vi "test-ltv-differential-drive-controller-Test1.vi"() -> (3 "All tests passed":bool)   [LabVIEW 2019]
uses:
  <vilib>/Rock Robotics/WPI/ThirdParty/JAS_Junk/TrajLib/TRAJ_STATE.ctl
  <vilib>/Rock Robotics/WPI/ThirdParty/JAS_Junk/TrajLib/POSE2D.ctl
  <vilib>/Rock Robotics/WPI/ThirdParty/JAS_Junk/TrajLib/TRANSLATION2D.ctl
  <vilib>/Rock Robotics/WPI/ThirdParty/JAS_Junk/TrajLib/ROTATION2D.ctl
  <vilib>/Rock Robotics/WPI/ThirdParty/JAS_Junk/TrajLib/LINEAR_SYSTEM.ctl
  <vilib>/Analysis/Matrix/Datatypes/RealMatrix.ctl
  <vilib>/Rock Robotics/WPI/ThirdParty/JAS_Junk/TrajLib/LTV_DIFF_DRIVE_CTRL.ctl
  <vilib>/Rock Robotics/WPI/ThirdParty/JAS_Junk/TrajLib/FUNCTION_GENERATOR_MATRIX.ctl
  <vilib>/Rock Robotics/WPI/ThirdParty/JAS_Junk/TrajLib/TRAJECTORY_SPLINE_TYPE_ENUM.ctl
  <vilib>/numeric/Random Number (Range) DBL.vi
  <vilib>/Rock Robotics/WPI/ThirdParty/JAS_Junk/TrajLib/Conv_Inches_Meters.vi
  <vilib>/Rock Robotics/WPI/ThirdParty/JAS_Junk/TrajLib/Rotation2d_CreateAngle.vi
  <vilib>/Rock Robotics/WPI/ThirdParty/JAS_Junk/TrajLib/Translation2d_Create.vi
  <vilib>/Rock Robotics/WPI/ThirdParty/JAS_Junk/TrajLib/MatBuilder_Create.vi
  <vilib>/Rock Robotics/WPI/ThirdParty/JAS_Junk/TrajLib/LinearSystem_New.vi
  <vilib>/Rock Robotics/WPI/ThirdParty/JAS_Junk/TrajLib/MatrixHelper_Zero.vi
  <vilib>/Rock Robotics/WPI/ThirdParty/JAS_Junk/TrajLib/MatBuilder_Fill.vi
  <vilib>/Rock Robotics/WPI/ThirdParty/JAS_Junk/TrajLib/SlewRateLimiter_New.vi
  <vilib>/Rock Robotics/WPI/ThirdParty/JAS_Junk/TrajLib/SlewRateLimiter_Reset.vi
  <vilib>/Rock Robotics/WPI/ThirdParty/JAS_Junk/TrajLib/SlewRateLimiter_Calculate.vi
  <vilib>/Rock Robotics/WPI/ThirdParty/JAS_Junk/TrajLib/SlewRateLimiter_SetRate.vi
  <vilib>/Rock Robotics/WPI/ThirdParty/JAS_Junk/TrajLib/MatrixHelper_CoerceSize.vi
  <vilib>/Rock Robotics/WPI/ThirdParty/JAS_Junk/TrajLib/Util_GetTime.vi
  <vilib>/Rock Robotics/WPI/ThirdParty/JAS_Junk/TrajLib/Trajectory_Library.lvlib
  <vilib>/Analysis/Matrix/NI_Matrix.lvlib
panel:
  out "DiffDriveCtrl":T1
  out "Output":T3
  out "Return X":T3
  out "Time":dbl=-1.0
  out "Create Error":bool
  out "Linearsystem":T4
  out "Error":bool
  out "IterationCount":i32
  out "Any Calc Error":bool
  out "Waveform Graph":dbl[][](graph)
  out "XY Graph":cluster{dbl[], dbl[]}[](graph)
  out "X":bool
  out "Y":bool
  out "Rot":bool
  out "TotalTime_Sec":dbl
  out "Calc Error":bool
  out "TrajStatePose":T5={"TRANSLATION"={"X"=0.0, "Y"=0.0}, "ROTATION"={"VALUE"=0.0, "COS"=1.0, "SIN"=0.0}} {"ROTATION"."SIN" format="%13.4f"; "ROTATION"."COS" format="%13.4f"; "ROTATION"."VALUE" format="%13.4f"; "TRANSLATION"."Y" format="%14.3f"; "TRANSLATION"."X" format="%14.3f"}
  out "UpdatedPose":T5 {"ROTATION"."SIN" format="%13.4f"; "ROTATION"."COS" format="%13.4f"; "ROTATION"."VALUE" format="%13.4f"; "TRANSLATION"."Y" format="%14.3f"; "TRANSLATION"."X" format="%14.3f"}
  out "OutputTRAJ_STATE":T8={"TimeSeconds"=0.0, "Velocity"=0.0, "Acceleration"=0.0, "POSE"={"TRANSLATION"={"X"=0.0, "Y"=0.0}, "ROTATION"={"VALUE"=0.0, "COS"=1.0, "SIN"=0.0}}, "Curvature"=0.0} {"POSE"."ROTATION"."SIN" format="%13.4f"; "POSE"."ROTATION"."COS" format="%13.4f"; "POSE"."ROTATION"."VALUE" format="%13.4f"; "POSE"."TRANSLATION"."Y" format="%14.3f"; "POSE"."TRANSLATION"."X" format="%14.3f"}
  out "At Reference":bool
  in  "Use Noise":bool
  in  "Use Rate Limit":bool
  # "< 5, 1 >"
  # "< 2 1 >"
  # "<States,States>"
  # "<States,Inputs>"
  # "<Outputs,States>"
  # "<Outputs,Inputs>"
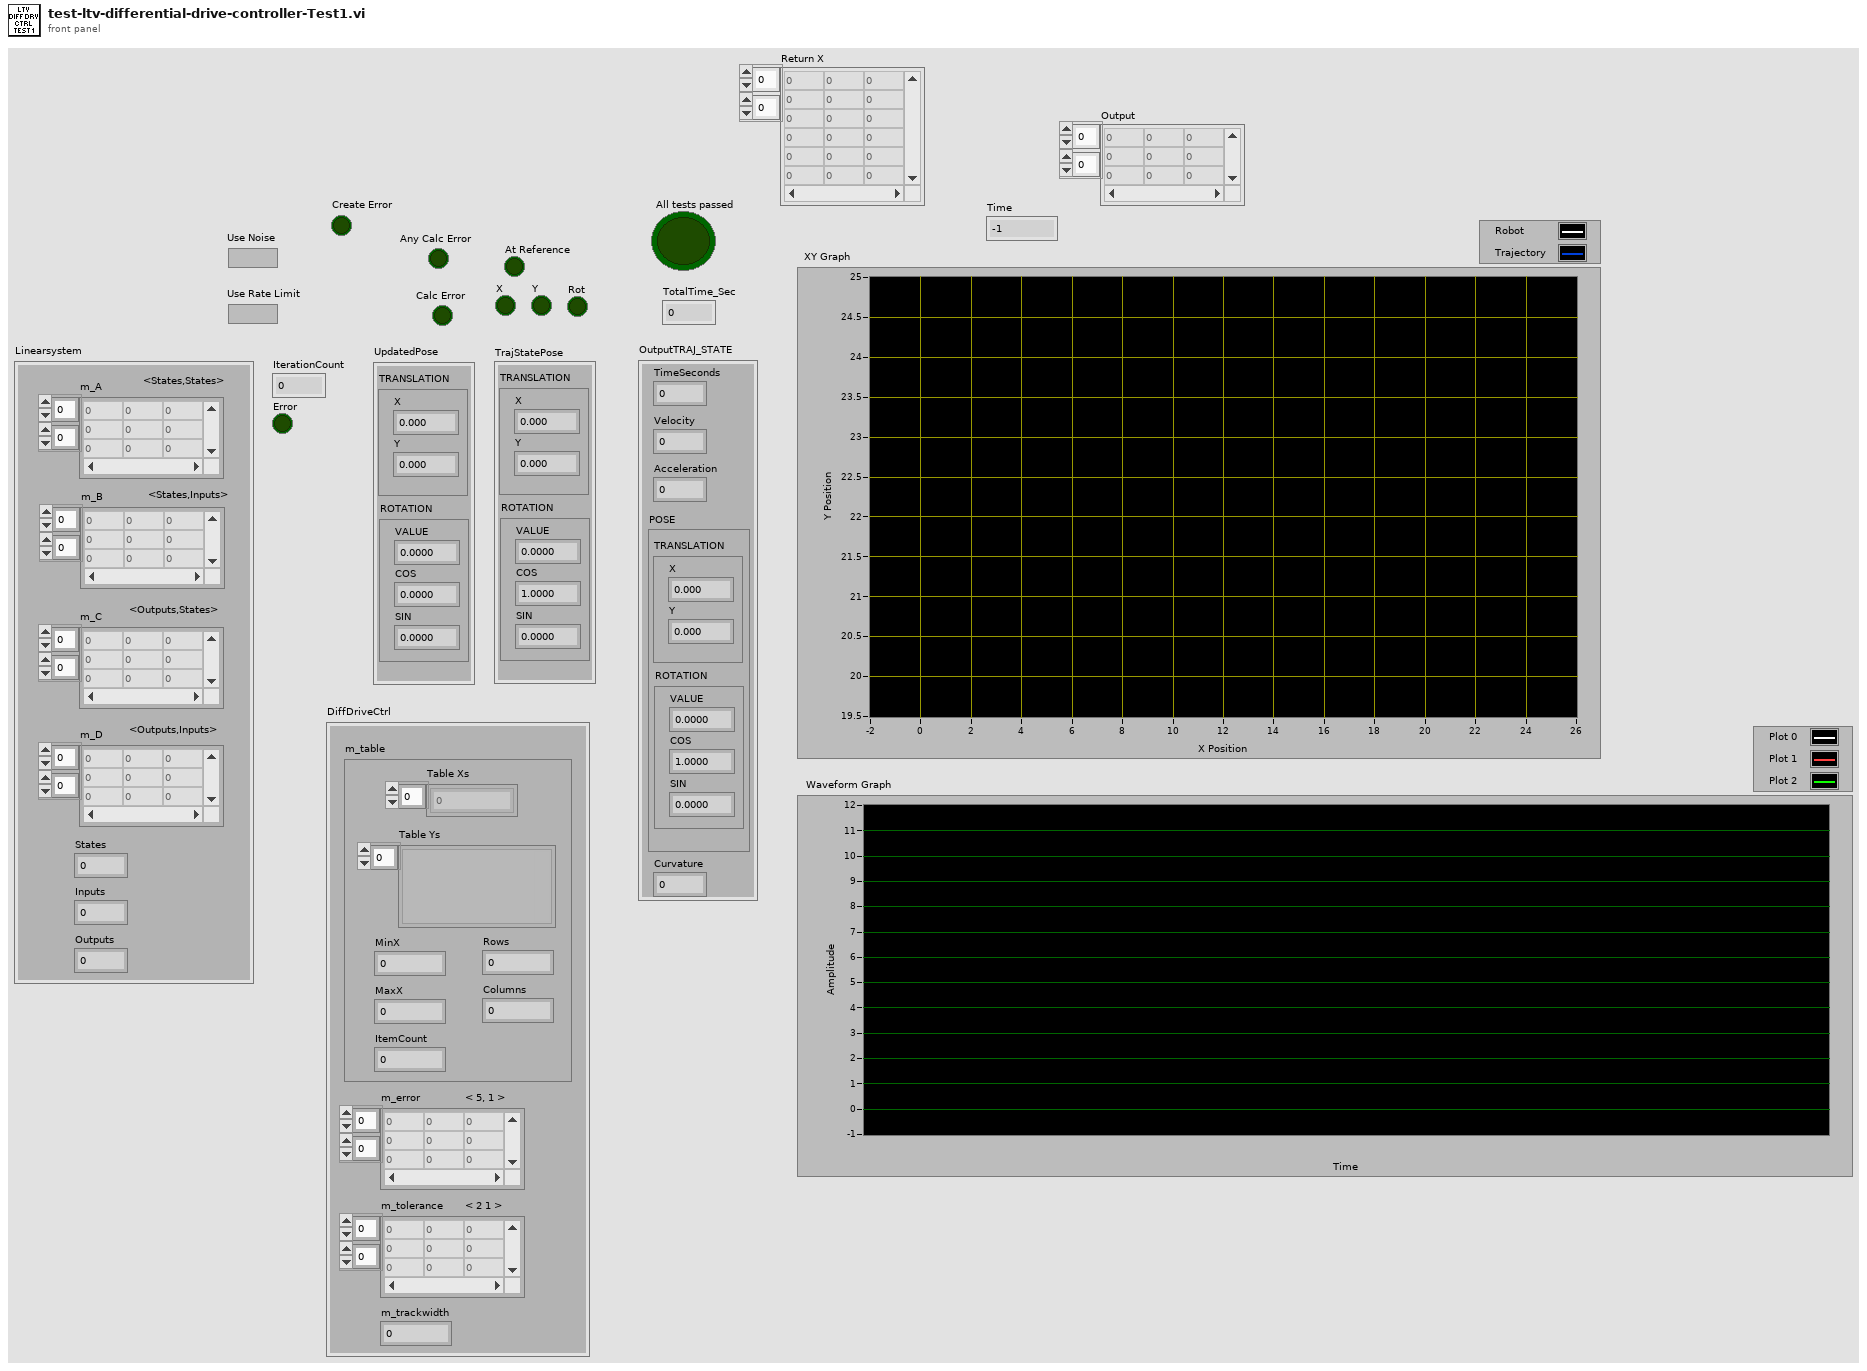
[diagram p1: front panel]
types:
  T1 = typedef "Trajectory_Library.lvlib/LTV_DIFF_DRIVE_CTRL.ctl" = cluster{"m_table":T2, "m_error":T3, "m_tolerance":T3, "m_trackwidth":dbl}
  T2 = typedef "Trajectory_Library.lvlib/FUNCTION_GENERATOR_MATRIX.ctl" = cluster{"Table Xs":dbl[], "Table Ys":variant[], "MinX":dbl, "MaxX":dbl, "ItemCount":i32, "Rows":i32, "Columns":i32}
  T3 = typedef "NI_Matrix.lvlib/RealMatrix.ctl" = dbl[][]
  T4 = typedef "Trajectory_Library.lvlib/LINEAR_SYSTEM.ctl" = cluster{"m_A":T3, "m_B":T3, "m_C":T3, "m_D":T3, "States":i32, "Inputs":i32, "Outputs":i32}
  T5 = typedef "Trajectory_Library.lvlib/POSE2D.ctl" = cluster{"TRANSLATION":T6, "ROTATION":T7}
  T6 = typedef "Trajectory_Library.lvlib/TRANSLATION2D.ctl" = cluster{"X":dbl, "Y":dbl}
  T7 = typedef "Trajectory_Library.lvlib/ROTATION2D.ctl" = cluster{"VALUE":dbl, "COS":dbl, "SIN":dbl}
  T8 = typedef "Trajectory_Library.lvlib/TRAJ_STATE.ctl" = cluster{"TimeSeconds":dbl, "Velocity":dbl, "Acceleration":dbl, "POSE":T5, "Curvature":dbl}
  T9 = typedef "Trajectory_Library.lvlib/TRAJECTORY_SPLINE_TYPE_ENUM.ctl" = enum16{"Cubic", "Cubic With Weights", "Quintic", "Quintic With Weights"}
  T10 = typedef "Trajectory_Library.lvlib/WEIGHTED_WAYPOINT.ctl" = cluster{"TRANSLATION":T6, "ROTATION":T7, "SCALAR":dbl}
  T11 = typedef "Trajectory_Library.lvlib/TRAJ_CONFIG.ctl" = cluster{"MaxVelocity":dbl, "Max Acceleration":dbl, "StartVelocity":dbl, "End Velocity":dbl, "Reversed":bool, "DiffDrKineConstntDefined":bool, "CentAcellConstntDefined":bool, "DiffDrVoltConstntDefined":bool, "DIFF_DRIVE_KINE_CONSTRAINT":T12, "CENTRIPETAL_ACCEL_CONSTRAINT":T14, "SwerveDrKineConstntDefined":bool, "SWERVE_DRIVE_KINE_CONSTRAINT":T15, "DIFF_DRIVE_VOLTAGE_CONSTRAINT":T17, "MECANUM_DRIVE_KINE_CONSTRAINT":T19, "MecanumDrKineConstntDefined":bool}
  T12 = typedef "Trajectory_Library.lvlib/TRAJ_CONSTRAINT_DIIF_DRIVE_KINEMATICS.ctl" = cluster{"Max Speed (M/S)":dbl, "DIFF_DRIVE_KINEMATICS":T13, "Max Accel (M/S2)":dbl}
  T13 = typedef "Trajectory_Library.lvlib/DIFF_DRIVE_KINEMATICS.ctl" = cluster{"TrackWidth_Meters":dbl}
  T14 = typedef "Trajectory_Library.lvlib/TRAJ_CONSTRAINT_CENTRIPETAL_ACCEL.ctl" = cluster{"Max Cent Accel":dbl}
  T15 = typedef "Trajectory_Library.lvlib/TRAJ_CONSTRAINT_SWERVE_DRIVE_KINEMATICS.ctl" = cluster{"Max Speed (M/S)":dbl, "SwerveKinematics":T16}
  T16 = typedef "Trajectory_Library.lvlib/SWERVE_DRIVE_KINEMATICS.ctl" = cluster{"NumModules":i32, "InverseKinematics":T3, "ForwardKinematics":T3, "Modules":T6[], "PrevCoR":T6}
  T17 = typedef "Trajectory_Library.lvlib/TRAJ_CONSTRAINT_DIIF_DRIVE_VOLTAGE.ctl" = cluster{"Max Voltage":dbl, "DIFF_DRIVE_KINEMATICS":T13, "SIMPLE_MOTOR_FF":T18}
  T18 = typedef "Trajectory_Library.lvlib/SIMPLE_MOTOR_FF.ctl" = cluster{"Ks":dbl, "Kv":dbl, "Ka":dbl}
  T19 = typedef "Trajectory_Library.lvlib/TRAJ_CONSTRAINT_MECA_DRIVE_KINEMATICS.ctl" = cluster{"Max Speed (M/S)":dbl, "MECA_DRIVE_KINEMATICS":T20}
  T20 = typedef "Trajectory_Library.lvlib/MECA_DRIVE_KINEMATICS.ctl" = cluster{"FrontLeft":T6, "FrontRight":T6, "RearLeft":T6, "RearRight":T6, "InverseKinematics":T3, "ForwardKinematics":T3, "PrevCoR":T6}
  T21 = typedef "Trajectory_Library.lvlib/TRAJECTORY.ctl" = cluster{"TotalTImeSecs":dbl, "States":T8[]}
  T22 = typedef "Trajectory_Library.lvlib/TWIST2D.ctl" = cluster{"dX":dbl, "dY":dbl, "dTHETA":dbl}
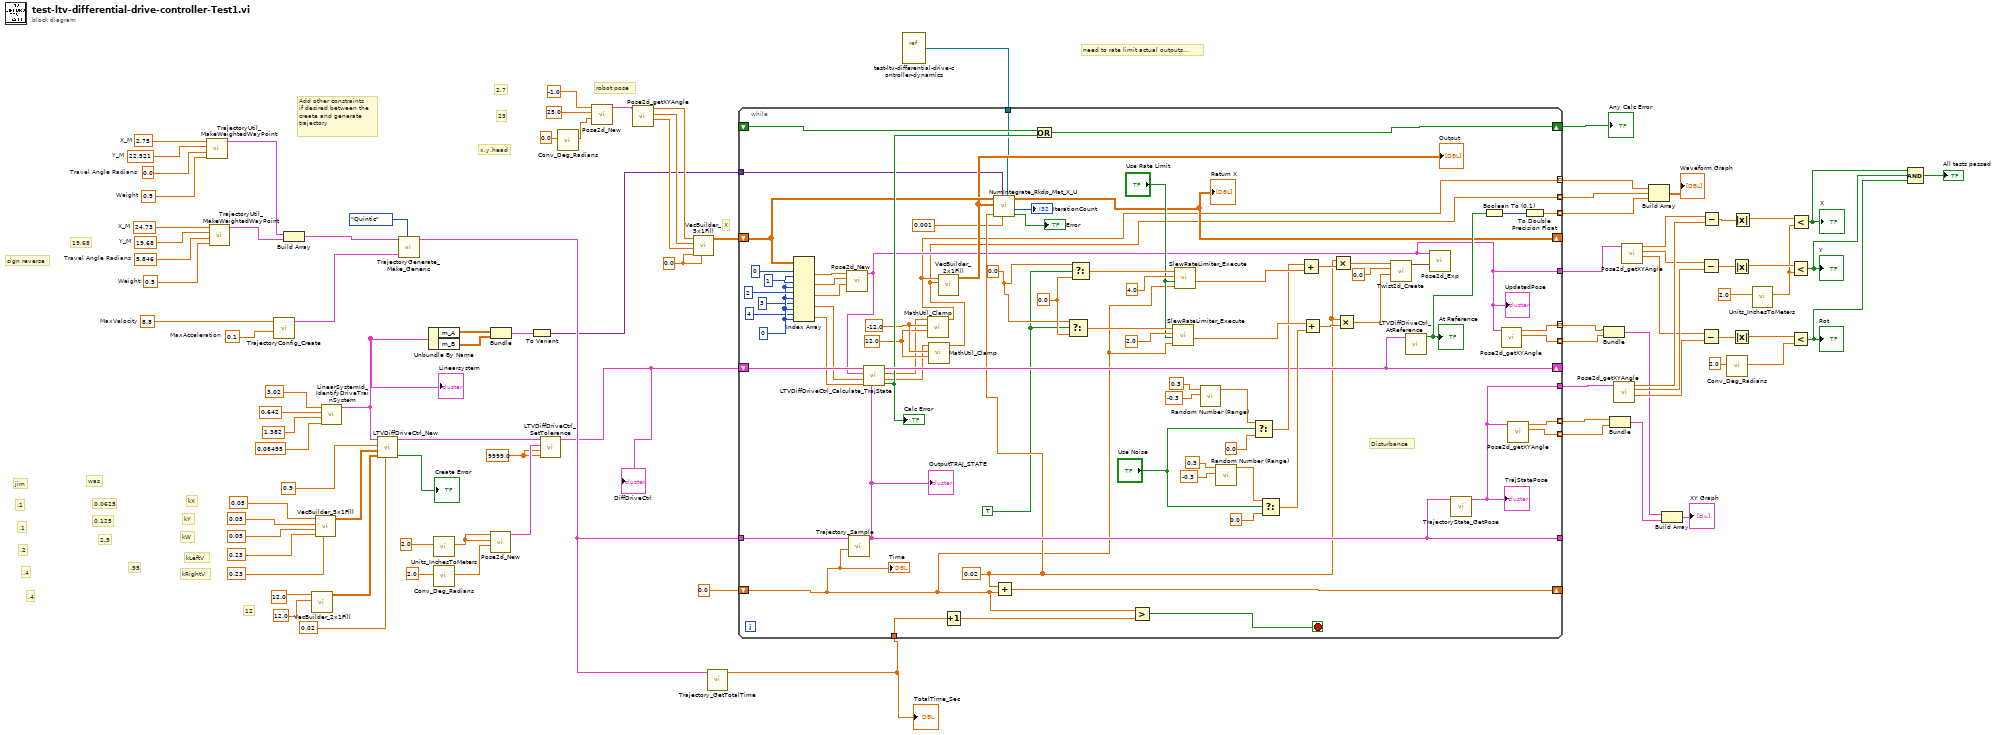
[diagram p0: block diagram]
diagram:
  w3 = 9999.0 ("LeftVelTolerance")
  w18 = 0.0 ("R3")
  w79 = 24.73  # X_M
  w78 = 19.68  # Y_M
  w66 = 5.846  # Travel Angle Radians
  w77 = 0.5  # Weight
  w76 = 2.75  # X_M
  w75 = 22.521  # Y_M
  w67 = 0.0  # Travel Angle Radians
  w74 = 0.5  # Weight
  w73 = 8.8  # MaxVelocity
  w72 = 0.1  # MaxAcceleration
  # ".4"
  # ".4"
  # ".2"
  # ".1"
  # ".1"
  # "jim"
  # "sign reverse"
  # "19.68"
  # ".95"
  # "12"
  # "need to rate limit actual outputs..."
  # "2.5"
  # "0.125"
  # "0.0625"
  # "was"
  # "X"
  # "23"
  # "2.7"
  # "x,y,head"
  # "robot pose"
  # "Add other constraints\nif desired between the\ncreate and generate\ntrajectory"
  # "kRightV"
  # "kLeftV"
  # "kW"
  # "kY"
  # "kX"
  n1 = call <vilib>:"TrajectoryUtil_MakeWeightedWayPoint.vi"("Weight"=w74, "Travel Angle Radians"=w67, "Y_M"=w75, "X_M"=w76) -> ("WEIGHTED_WAYPOINT"=w68:T10)  [unwired: 7 in]
  n2 = call <vilib>:"TrajectoryUtil_MakeWeightedWayPoint.vi"("Weight"=w77, "Travel Angle Radians"=w66, "Y_M"=w78, "X_M"=w79) -> ("WEIGHTED_WAYPOINT"=w80:T10)  [unwired: 7 in]
  n3 = call <vilib>:"TrajectoryConfig_Create.vi"("MaxAcceleration"=w72, "MaxVelocity"=w73) -> ("TRAJECTORY_CONFIG"=w71:T11)  [unwired: 9 in]
  n4 = Build Array(w68, w80) -> (w69:T10[])
  n5 = call <vilib>:"VecBuilder_2x1Fill.vi"("R1"=12.0, "R0"=12.0) -> ("output matrix"=w59:T3)  [unwired: 9 in]
  n6 = call <vilib>:"VecBuilder_5x1Fill.vi"("R4"=0.23, "R3"=0.23, "R2"=0.05, "R1"=0.05, "R0"=0.05) -> ("output matrix"=w60:T3)  [unwired: 6 in]
  n7 = call <vilib>:"LinearSystemId_IdentifyDriveTrainSystem.vi"("kAAngular"=0.08495, "kVAngular"=1.382, "kALinear"=0.642, "kVLinear"=3.02) -> ("Linearsystem"=w12:T4)  [unwired: 6 in, 1 out]
  "Linearsystem" <- w12
  n8 = call <vilib>:"LTVDiffDriveCtrl_New.vi"("dT"=0.02, "Relms"=w59, "Qelms"=w60, "TrackWidth"=0.9, "Plant"=w12) -> ("Error"=→"Create Error":bool, "DiffDriveCtrl"=w6:T1)  [unwired: 5 in]
  n9 = call <vilib>:"TrajectoryGenerate_Make_Generic.vi"("Spline Type"=TRAJECTORY_SPLINE_TYPE_ENUM."Quintic", "traj_config"=w71, "WeightedWayPoints"=w69) -> ("TRAJECTORY"=w56:T21)  [unwired: 7 in, 1 out]
  n10 = Unbundle By Name(w12) -> ("m_A"=w16:T3, "m_B"=w15:T3)
  n11 = call <vilib>:"Units_InchesToMeters.vi"("Inches"=2.0 ("x")) -> ("Meters"=w8:dbl)  [unwired: 10 in]
  n12 = call <vilib>:"Conv_Deg_Radians.vi"("Degress"=2.0) -> ("Radians"=w7:dbl)  [unwired: 10 in]
  n13 = call <vilib>:"Pose2d_New.vi"("Heading"=w7, "Y"=w8, "X"=w8) -> ("out POSe"=w4:T5)  [unwired: 8 in]
  n14 = Bundle("m_A"=w16, "m_B"=w15) -> (w14:cluster{"m_A":T3, "m_B":T3})  [unwired: 1 in]
  n15 = To Variant(anything=w14) -> (Variant=w13:variant)
  n16 = call <vilib>:"LTVDiffDriveCtrl_SetTolerance.vi"("RightVelTolerance"=w3, "LeftVelTolerance"=w3, "PoseTolerance"=w4, "in LTV_DIFF_DRIVE_CONTROLLER"=w6) -> ("out LTV_DIFF_DRIVE_CONTROLLER"=w5:T1)  [unwired: 7 in]
  "DiffDriveCtrl" <- w5
  n17 = call <vilib>:"Conv_Deg_Radians.vi"("Degress"=0.0) -> ("Radians"=w65:dbl)  [unwired: 10 in]
  n18 = call <vilib>:"Pose2d_New.vi"("Heading"=w65, "Y"=25.0, "X"=-1.0) -> ("out POSe"=w23:T5)  [unwired: 8 in]
  n19 = call <vilib>:"Pose2d_getXYAngle.vi"("in POSE"=w23) -> ("Angle"=w19:dbl, "Y"=w20:dbl, "X"=w21:dbl)  [unwired: 8 in]
  n20 = call <vilib>:"VecBuilder_5x1Fill.vi"("R4"=w18, "R3"=w18, "R2"=w19, "R1"=w20, "R0"=w21) -> ("output matrix"=w22:T3)  [unwired: 6 in]
  n21 = call <vilib>:"Trajectory_GetTotalTime.vi"("TRAJECTORY"=w56) -> ("TotalTime_Sec"=w57:dbl)  [unwired: 10 in]
  "TotalTime_Sec" <- w57
  n22 = vi-ref "test-ltv-differential-drive-controller-dynamics.vi"() -> (w17:refnum<vi>)
  n23 = while {
    shift-right: [w165] -> _
    shift-left: 0.0 -> [w94]
    tunnel: w57 -> [w128]
    tunnel: w56 -> [w164]
    shift-right: [w110] -> _
    shift-left: w22 -> [w111]
    shift-right: [w125] -> _
    shift-left: w5 -> [w126]
    tunnel: [w124] -> _
    tunnel: [w155] -> w30
    tunnel: [w159] -> w29 mode=indexing
    tunnel: [w158] -> w28 mode=indexing
    tunnel: [w157] -> w31 mode=indexing
    tunnel: [w156] -> w32 mode=indexing
    tunnel: [w104] -> w24
    tunnel: [w150] -> w27 mode=indexing
    shift-right: [w140] -> w26
    shift-left: _ -> [w141]
    tunnel: w17 -> [w103]
    tunnel: w13 -> [w102]
    tunnel: [w96] -> w2 mode=indexing
    tunnel: [w95] -> w1 mode=indexing
    stop <- w166 stop-if-true
    w93 = TRUE
    w99 = 12.0 ("High Limit")
    w100 = -12.0 ("Low Limit")
    w105 = 0.0 ("t")
    w117 = 0 ("index (col)")
    w130 = 0.0 ("f")
    w109 = 0.02 ("x")
    # "Disturbance"
    n24 = Index Array(array=w111, index (row) #1=0 ("index (row)"), index (col) #1=w117, index (row) #2=1 ("index (row)"), index (col) #2=w117, index (row) #3=2 ("index (row)"), index (col) #3=w117, index (row) #4=3 ("index (row)"), index (col) #4=w117, index (row) #5=4 ("index (row)"), index (col) #5=w117) -> (element #1=w120:dbl, element #2=w119:dbl, element #3=w118:dbl, element #4=w114:dbl, element #5=w113:dbl)
    n25 = call <vilib>:"Pose2d_New.vi"("Heading"=w118, "Y"=w119, "X"=w120) -> ("out POSe"=w104:T5)  [unwired: 8 in]
    "UpdatedPose" <- w104
    n26 = call <vilib>:"Trajectory_Sample.vi"("Time"=w94, "InputTRAJECTORY"=w164) -> ("OutputTRAJ_STATE"=w124:T8)  [unwired: 9 in]
    "OutputTRAJ_STATE" <- w124
    n27 = call <vilib>:"LTVDiffDriveCtrl_Calculate_TrajState.vi"("DesiredState"=w124, "Right Velocity"=w113, "Left Velocity"=w114, "CurrentPose"=w104, "in LTVDiffDrveCtrl"=w126) -> ("Error"=w112:bool, "Right Voltage"=w97:dbl, "Left Voltage"=w98:dbl, "out LTVDiffDriveCtrl"=w125:T1)  [unwired: 3 in]
    "Calc Error" <- w112
    n28 = call <vilib>:"MathUtil_Clamp.vi"("High Limit"=w99, "Low Limit"=w100, "Value"=w98) -> ("Result"=w96:dbl)  [unwired: 8 in]
    n29 = call <vilib>:"MathUtil_Clamp.vi"("High Limit"=w99, "Low Limit"=w100, "Value"=w97) -> ("Result"=w95:dbl)  [unwired: 8 in]
    n30 = call <vilib>:"VecBuilder_2x1Fill.vi"("R1"=w95, "R0"=w96) -> ("output matrix"=w108:T3)  [unwired: 9 in]
    "Output" <- w108
    n31 = Increment(x=w128) -> (x+1=w127:dbl)
    n32 = call <vilib>:"NumIntegrate_Rkdp_Mat_X_U.vi"("Func_X_U_Extra"=w103, "MaxError"=0.001, "PassedData"=w102, "dT_Seconds"=w109, "U"=w108, "X"=w111) -> ("Error"=→"Error":bool, "IterationCount"=→"IterationCount":i32, "Return X"=w110:T3)  [unwired: 3 in]
    "Return X" <- w110
    n33 = Add(x=w109, y=w94) -> (x+y=w165:dbl)
    n34 = Or(x=w141, y=w112) -> (x .or. y?=w140:bool)
    n35 = Select(t=w105, s=w93, f=w130) -> (s? t:f=w132:dbl)
    n36 = Select(t=w105, s=w93, f=w130) -> (s? t:f=w131:dbl)
    n37 = Greater?(x=w94, y=w127) -> (0:w166:bool)
    n38 = call <vilib>:"SlewRateLimiter_Execute.vi"("Time"=w94, "Enable"="Use Rate Limit", "Rate"=2.0, "Input"=w132) -> ("Output"=w149:dbl)  [unwired: 6 in, 1 out]
    n39 = call <vilib>:"SlewRateLimiter_Execute.vi"("Time"=w94, "Enable"="Use Rate Limit", "Rate"=4.0, "Input"=w131) -> ("Output"=w147:dbl)  [unwired: 6 in, 1 out]
    n40 = call-poly <vilib>:"Random Number (Range).vi"("lower bound (0)"=-0.3, "upper bound (100)"=0.3) -> ("number"=w137:dbl)  [unwired: 9 in]
    n41 = call-poly <vilib>:"Random Number (Range).vi"("lower bound (0)"=-0.3, "upper bound (100)"=0.3) -> ("number"=w134:dbl)  [unwired: 9 in]
    n42 = Select(t=w137, s="Use Noise", f=0.0) -> (s? t:f=w139:dbl)
    n43 = Select(t=w134, s="Use Noise", f=0.0) -> (s? t:f=w135:dbl)
    n44 = Add(x=w139, y=w147) -> (x+y=w146:dbl)
    n45 = Add(x=w149, y=w135) -> (x+y=w148:dbl)
    n46 = Multiply(x=w109, y=w146) -> (x*y=w162:dbl)
    n47 = Multiply(x=w109, y=w148) -> (x*y=w160:dbl)
    n48 = call <vilib>:"Twist2d_Create.vi"("dTHETA"=w160, "dY"=0.0, "dX"=w162) -> ("TWIST"=w163:T22)  [unwired: 8 in]
    n49 = call <vilib>:"LTVDiffDriveCtrl_AtReference.vi"("LTV_DIFF_DRIVE_CTRL"=w125) -> ("At Reference"=w152:bool)  [unwired: 10 in]
    "At Reference" <- w152
    n50 = call <vilib>:"Pose2d_Exp.vi"("TWIST"=w163, "POSE"=w104) -> ()  [unwired: 9 in, 1 out]
    n51 = call <vilib>:"TrajectoryState_GetPose.vi"("TRAJ_STATE"=w124) -> ("TrajStatePose"=w155:T5)  [unwired: 10 in]
    "TrajStatePose" <- w155
    n52 = Boolean To (0,1)(Boolean=w152) -> (0, 1=w151:i16)
    n53 = call <vilib>:"Pose2d_getXYAngle.vi"("in POSE"=w104) -> ("Y"=w158:dbl, "X"=w159:dbl)  [unwired: 8 in, 1 out]
    n54 = call <vilib>:"Pose2d_getXYAngle.vi"("in POSE"=w155) -> ("Y"=w156:dbl, "X"=w157:dbl)  [unwired: 8 in, 1 out]
    n55 = To Double Precision Float(number=w151) -> (double precision float=w150:dbl)
    "Time" <- w94
  }
  "Any Calc Error" <- w26
  n56 = Bundle(w29, w28) -> (w41:cluster{dbl[], dbl[]})  [unwired: 1 in]
  n57 = Bundle(w31, w32) -> (w40:cluster{dbl[], dbl[]})  [unwired: 1 in]
  n58 = call <vilib>:"Pose2d_getXYAngle.vi"("in POSE"=w30) -> ("Angle"=w44:dbl, "Y"=w46:dbl, "X"=w52:dbl)  [unwired: 8 in]
  n59 = call <vilib>:"Pose2d_getXYAngle.vi"("in POSE"=w24) -> ("Angle"=w45:dbl, "Y"=w47:dbl, "X"=w53:dbl)  [unwired: 8 in]
  n60 = Build Array(w2, w1, w27) -> (→"Waveform Graph":dbl[][])
  n61 = Build Array(w41, w40) -> (→"XY Graph":cluster{dbl[], dbl[]}[])
  n62 = Subtract(x=w47, y=w46) -> (x-y=w50:dbl)
  n63 = Subtract(x=w45, y=w44) -> (x-y=w48:dbl)
  n64 = Subtract(x=w53, y=w52) -> (x-y=w54:dbl)
  n65 = call <vilib>:"Conv_Deg_Radians.vi"("Degress"=2.0) -> ("Radians"=w42:dbl)  [unwired: 10 in]
  n66 = Absolute Value(x=w50) -> (abs(x)=w51:dbl)
  n67 = Absolute Value(x=w48) -> (abs(x)=w49:dbl)
  n68 = Absolute Value(x=w54) -> (abs(x)=w55:dbl)
  n69 = call <vilib>:"Units_InchesToMeters.vi"("Inches"=2.0 ("x")) -> ("Meters"=w34:dbl)  [unwired: 10 in]
  n70 = Less?(x=w51, y=w34) -> (x < y?=w36:bool)
  "Y" <- w36
  n71 = Less?(x=w49, y=w42) -> (x < y?=w35:bool)
  "Rot" <- w35
  n72 = Less?(x=w55, y=w34) -> (x < y?=w37:bool)
  "X" <- w37
  n73 = Compound Arithmetic op=AND(w37, w36, w35) -> (→"All tests passed":bool)
